vi "smart door working keypad myrio version.vi"() -> ()   [LabVIEW 2017]
uses:
  <vilib>/myRIO/Instrument Drivers/Onboard IO/DIO/typedefs/DIO Reference.ctl
  <vilib>/myRIO/Common/Instrument Driver Framework/Utilities/typedefs/myRIO Generic Hardware Reference.ctl
  <vilib>/myRIO/Common/Instrument Driver Framework/Utilities/typedefs/Hardware Version Enum.ctl
  <vilib>/myRIO/Common/Instrument Driver Framework/Utilities/typedefs/myRIO v1.0 Reference.ctl
  <vilib>/myRIO/Common/Instrument Driver Framework/Utilities/typedefs/Generic FPGA Reference.ctl
  <vilib>/myRIO/Common/Instrument Driver Framework/myRIO v1.0/DIO/typedefs/DIO Channels List.ctl
  <vilib>/myRIO/Common/Instrument Driver Framework/myRIO v1.0/DIO/typedefs/DIO Channels Enum.ctl
  <vilib>/userdefined/High Color/nirio_resource_hc.ctl
  <vilib>/myRIO/Common/Instrument Driver Framework/Utilities/vis/Is FPGA Ref Available.vi
  <vilib>/myRIO/Common/Instrument Driver Framework/myRIO v1.0/DIO/vis/myRIO v1.1 Open DIO.vi
  <vilib>/myRIO/Instrument Drivers/Onboard IO/DIO/vis/Write.vi
  <vilib>/myRIO/Common/Instrument Driver Framework/Utilities/vis/Validate Channels.vi
  <vilib>/myRIO/Common/Instrument Driver Framework/myRIO v1.0/DIO/vis/myRIO v1.0 Reserve DIO.vi
  <vilib>/myRIO/Common/Instrument Driver Framework/myRIO v1.0/Resource Manager/vis/myRIO v1.0 Reserve Channel List.vi
  <vilib>/myRIO/Common/Instrument Driver Framework/myRIO v1.0/DIO/vis/myRIO v1.0 Build MUX Configuration DIO.vi
  <vilib>/myRIO/Common/Instrument Driver Framework/myRIO v1.0/Resource Manager/vis/myRIO v1.0 Reserve Channel.vi
  <vilib>/myRIO/Common/Instrument Driver Framework/myRIO v1.0/Resource Manager/vis/myRIO v1.0 Unreserve Channel.vi
  <vilib>/myRIO/Common/Instrument Driver Framework/myRIO v1.0/Resource Manager/vis/myRIO v1.0 Create Configuration List.vi
  <vilib>/myRIO/Common/Instrument Driver Framework/myRIO v1.0/Resource Manager/vis/myRIO v1.0 Build Mutex Name.vi
  <vilib>/Utility/VariantDataType/GetNumericInfo.vi
  <vilib>/Utility/error.llb/Error Cluster From Error Code.vi
  <vilib>/myRIO/Common/Instrument Driver Framework/myRIO v1.0/myRIO v1.1 Open.vi
  <vilib>/myRIO/Common/Instrument Driver Framework/Utilities/vis/IO Manager.vi
  <vilib>/myRIO/Common/Instrument Driver Framework/Utilities/vis/Configuration Manager.vi
  <vilib>/myRIO/Common/Instrument Driver Framework/myRIO v1.0/Resource Manager/vis/myRIO v1.0 Configure IO.vi
  <vilib>/myRIO/Common/Instrument Driver Framework/myRIO v1.0/myRIO v1.0 Close.vi
  <vilib>/myRIO/Common/Instrument Driver Framework/myRIO v1.0/DIO/vis/myRIO v1.0 Write DIO.vi
  <vilib>/myRIO/Express VI/Onboard Devices/LED/LED Express VI.xnode
  <vilib>/myRIO/Instrument Drivers/Onboard IO/DIO/vis/myRIO DIO Open.xnode
  <vilib>/myRIO/Instrument Drivers/Onboard IO/DIO/DIO.lvlib
panel:
  out "Boolean 3":bool
  out "Boolean 2":bool
  in  "stop":bool
  out "Boolean":bool
  in  "?":bool
  in  "?":bool
  in  "?":bool
  in  "?":bool
  in  "?":bool
  in  "?":bool
  in  "?":bool
  in  "?":bool
  in  "?":bool
  in  "?":bool
  in  "Enter":bool
  out "Passcode (4 Ditgits)":string
  out "Wrong":bool
  out "Correct":bool
  out "String 2":string
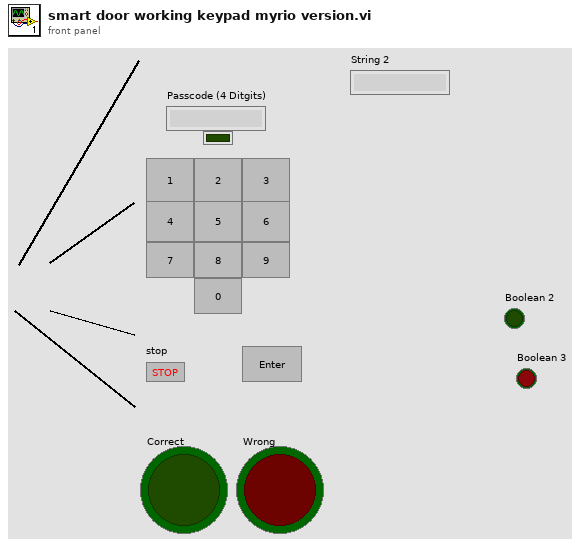
[diagram p1: front panel]
types:
  T1 = typedef "DIO.lvlib/DIO Reference.ctl" = cluster{"myRIO Reference":T2, "DIO Channels List":T6}
  T2 = typedef "myRIO Generic Hardware Reference.ctl" = cluster{"myRIO Model":T3, "myRIO Hardware Reference":T4}
  T3 = typedef "Hardware Version Enum.ctl" = enum16{"Unknown", "myRIO-1900", "myRIO-1950", "roboRIO", "NI ELVIS RIO CM"}
  T4 = typedef "myRIO v1.0 Reference.ctl" = cluster{"Generic FPGA Reference":T5, "Allow multiple opens":bool}
  T5 = typedef "Generic FPGA Reference.ctl" = refnum<k20>
  T6 = typedef "DIO Channels List.ctl" = T7[]
  T7 = typedef "DIO Channels Enum.ctl" = enum16{"Not Connected", "C/DIO0", "C/DIO1", "C/DIO2", "C/DIO3", "C/DIO4", "C/DIO5", "C/DIO6", "C/DIO7", "A/DIO0", "A/DIO1", "A/DIO2", "A/DIO3", "A/DIO4", "A/DIO5", "A/DIO6", "A/DIO7", "A/DIO8", "A/DIO9", "A/DIO10", "A/DIO11", "A/DIO12", "A/DIO13", "A/DIO14", "A/DIO15", "B/DIO0", "B/DIO1", "B/DIO2", "B/DIO3", "B/DIO4", "B/DIO5", "B/DIO6", "B/DIO7", "B/DIO8", "B/DIO9", "B/DIO10", "B/DIO11", "B/DIO12", "B/DIO13", "B/DIO14", "B/DIO15", "LED0", "LED1", "LED2", "LED3", "Button0", "DIO/DIO0", "DIO/DIO1", "DIO/DIO2", "DIO/DIO3", "DIO/DIO4", "DIO/DIO5", "DIO/DIO6", "DIO/DIO7", "DIO/DIO8", "DIO/DIO9", "SPI/CS0", "SPI/CS1", "SPI/CS2", "SPI/CS3", "LED RADIO (Green)", "LED RADIO (Red)", "LED COMM (Green)", "LED COMM (Red)", "LED MODE (Green)", "LED MODE (Red)"}
  T8 = typedef "nirio_resource_hc.ctl" = tag
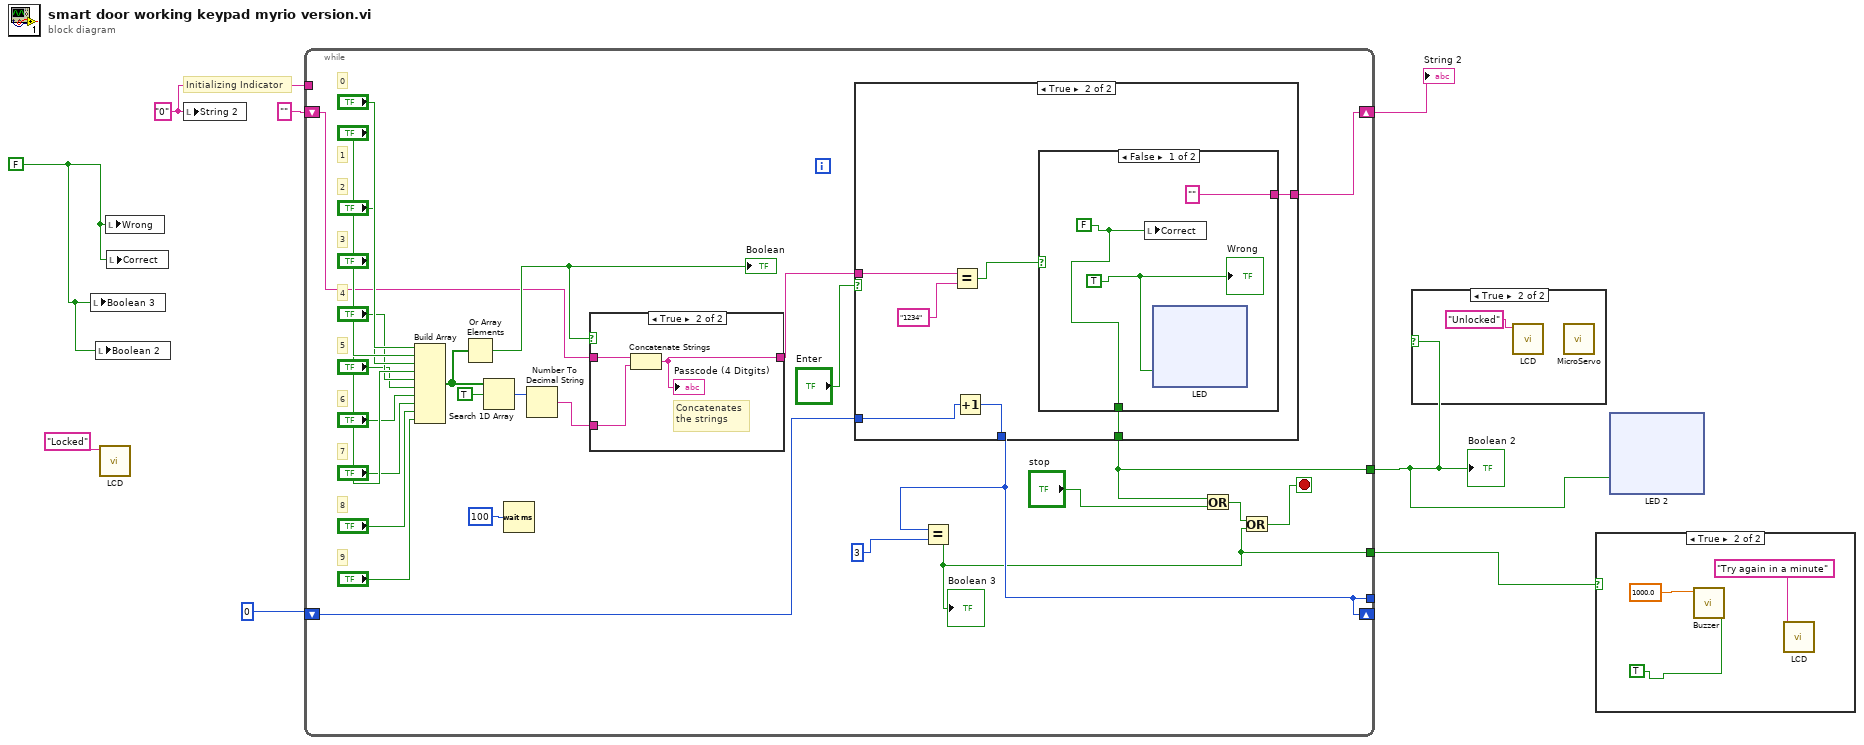
[diagram p0: block diagram]
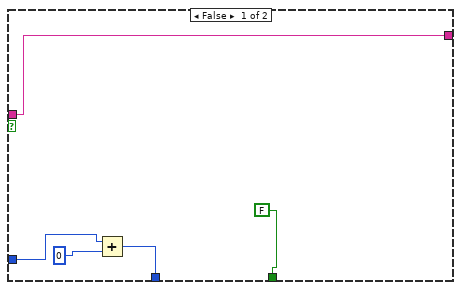
[diagram p4: hidden frame]
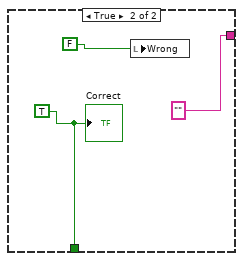
[diagram p5: hidden frame]
diagram:
  w4 = FALSE
  w7 = "0" ("String")
  # "Initializing Indicator"
  n1 = local write "Boolean 3"(w4) -> ()
  n2 = local write "Boolean 2"(w4) -> ()
  n3 = call "LCD.vi"("String"="Locked") -> ()  [unwired: 11 in]
  n4 = local write "Wrong"(w4) -> ()
  n5 = local write "Correct"(w4) -> ()
  n6 = local write "String 2"(w7) -> ()
  n7 = while {
    shift-right: [w17] -> w6
    shift-left: "" -> [w21]
    tunnel: w7 -> [_]
    tunnel: [w15] -> w3
    shift-right: [w13] -> _
    shift-left: 0 -> [w14]
    tunnel: [w13] -> _
    tunnel: [w9] -> w2
    stop <- w10 stop-if-true
    # "9"
    # "8"
    # "7"
    # "6"
    # "5"
    # "4"
    # "3"
    # "2"
    # "1"
    # "0"
    n8 = Build Array("?", "?", "?", "?", "?", "?", "?", "?", "?", "?") -> (w35:bool[])
    n9 = Or Array Elements(Boolean array=w35) -> (logical OR=w22:bool)
    "Boolean" <- w22
    n10 = Search 1D Array(1D array=w35, element=TRUE) -> (index of element=w36:i32)  [unwired: 1 in]
    n11 = Wait (ms)(milliseconds to wait=u32 100) -> ()  [unwired: 1 out]
    n12 = Number To Decimal String(number=w36) -> (decimal integer string=w23:string)  [unwired: 1 in]
    n13 = case shown="True" w22 {
      tunnel: w23 -> [_ w92]
      tunnel: w21 -> [w90 w93]
      tunnel: [w90 w91] -> w18
      frame False {
        # "if no buttons pressed\n-1 is ignored."
      }
      frame True {
        # "Concatenates\nthe strings"
        n14 = Concatenate Strings(w93, w92) -> (w91:string)
        "Passcode (4 Ditgits)" <- w91
      }
    }
    n15 = case shown="True" "Enter" {
      tunnel: w18 -> [w41 w46]
      tunnel: [w41 w45] -> w17
      tunnel: [FALSE w44] -> w15
      tunnel: w14 -> [w38 w43]
      tunnel: [w37 w42] -> w13
      frame False {
        n16 = Add(x=w38, y=0) -> (x+y=w37:i32)
      }
      frame True {
        n17 = Equal?(x=w46, y="1234") -> (x = y?=w48:bool)
        n18 = Increment(x=w43) -> (x+1=w42:i32)
        n19 = case shown="False" w48 {
          tunnel: ["" ""] -> w45
          tunnel: [w50 w87] -> w44
          frame False {
            w49 = TRUE
            w50 = FALSE
            n20 = local write "Correct"(w50) -> ()
            n21 = xnode "LED"("RED"=w49) -> ()  [unwired: 1 in, 1 out]
            "Wrong" <- w49
          }
          frame True {
            w87 = TRUE
            n22 = local write "Wrong"(FALSE) -> ()
            "Correct" <- w87
          }
        }
      }
    }
    n23 = Equal?(x=w13, y=3) -> (x = y?=w9:bool)
    "Boolean 3" <- w9
    n24 = Or(x=w15, y="stop") -> (x .or. y?=w11:bool)
    n25 = Or(x=w11, y=w9) -> (x .or. y?=w10:bool)
  }
  "String 2" <- w6
  "Boolean 2" <- w3
  n26 = case shown="True" w3 {
    frame False {
    }
    frame True {
      n27 = call "LCD.vi"("String"="Unlocked") -> ()  [unwired: 11 in]
      n28 = call "MicroServo.vi"() -> ()  [unwired: 12 in]
    }
  }
  n29 = case shown="True" w2 {
    frame False {
    }
    frame True {
      n30 = call "Buzzer.vi"("[ESC]"=TRUE, "frequency [Hz]"=1000.0) -> ()  [unwired: 10 in]
      n31 = call "LCD.vi"("String"="Try again in a minute") -> ()  [unwired: 11 in]
    }
  }
  n32 = xnode "LED 2"("Green"=w3) -> ()  [unwired: 1 in, 1 out]
